vi "Modbus_Slave.vi"() -> ()   [LabVIEW 2020]
uses:
  <vilib>/NI/Modbus Library/API/Wrapper/Create TCP Slave.vi
  <vilib>/NI/Modbus Library/API/Slave/Modbus Slave.lvclass
  <vilib>/NI/Modbus Library/API/Wrapper/API Main.lvlib
panel:
  out "Array":u16[](array[knob]) scale=0.0..100.0
  in  "starting address":u16
  in  "number of inputs":u16
  in  "stop":bool
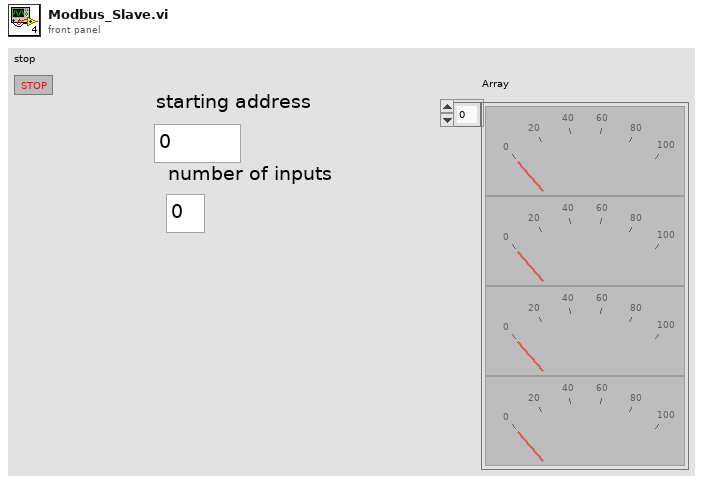
[diagram p1: front panel]
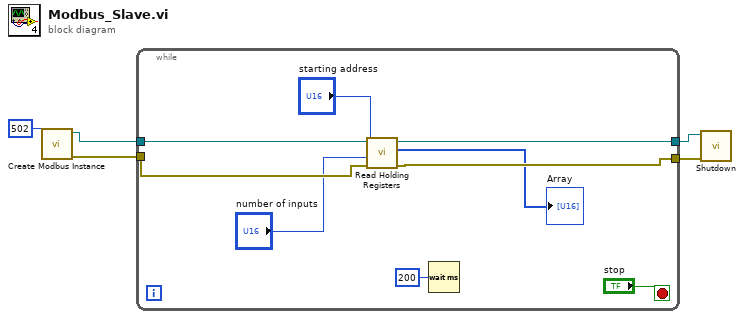
[diagram p0: block diagram]
diagram:
  n1 = call-poly <vilib>:"Create Modbus Instance.vi"("port (502)"=u16 502) -> ("error out"=w2:errorcluster, "TCP slave instance"=w5:refnum<class "Modbus Slave.lvclass">)  [unwired: 9 in]
  n2 = while {
    tunnel: w5 -> [w12]
    tunnel: [w11] -> w4
    tunnel: [w10] -> w3
    tunnel: w2 -> [w9]
    stop <- "stop" stop-if-true
    n3 = call-dynamic "Read Holding Registers.vi"("error in"=w9, "number of inputs"="number of inputs", "starting address"="starting address", "Modbus slave in"=w12) -> ("error out"=w10:errorcluster, "register values"=→"Array":u16[], "Modbus slave out"=w11:refnum<class "Modbus Slave.lvclass">)  [unwired: 5 in]
    n4 = Wait (ms)(milliseconds to wait=u32 200) -> ()  [unwired: 1 out]
  }
  n5 = call-dynamic "Shutdown.vi"("error in"=w3, "Modbus slave in"=w4) -> ()  [unwired: 9 in, 1 out]
